vi "9401_UI.vi"(8 "error in (no error)":errorcluster, 11 "Node Ptr":T1 format="%.0x") -> (0 "error out":errorcluster)   [LabVIEW 2019, in "Modules.lvlib" / "9401.lvclass"]
uses:
  9401.lvclass
  <vilib>/NI VeriStand/Custom Device API/Custom Device Item Ref.ctl
  RSI Module/SubPanel Command.ctl
  C:/Users/nitest/Desktop/Git 2019/niveristand-scan-engine-module-libraries/Source/RSI Module/RSI Module.lvclass
  9401.lvclass/9401.ctl
  RSI Module/RSI Module.lvclass
  <vilib>/NI VeriStand/Custom Device API/Custom Device API.lvlib
panel:
  out "_Initial Line Direction Label":string="Initial Line Direction"
  in  "DIO3:0":u32(ring) items=["Input", "Output"]
  in  "DIO7:4":u32(ring) items=["Input", "Output"]
  in  "SubPanel Event":refnum<user-event>
  in  "Header":cluster{"Section Name":string}={"Section Name"="NI 9205 Settings"}
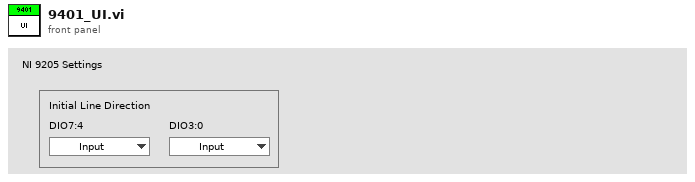
[diagram p1: front panel]
types:
  T1 = typedef "Custom Device API.lvlib/Custom Device Item Ref.ctl" = u64
  T2 = typedef "Modules.lvlib/RSI Module.lvclass/Module Models.ctl" = enum16{"Empty", "NI 9201", "NI 9203", "NI 9205", "NI 9206", "NI 9207", "NI 9208", "NI 9209", "NI 9210", "NI 9211", "NI 9212", "NI 9213", "NI 9214", "NI 9215", "NI 9216", "NI 9217", "NI 9219", "NI 9220", "NI 9221", "NI 9222", "NI 9223", "NI 9224", "NI 9225", "NI 9226", "NI 9227", "NI 9228", "NI 9229", "NI 9233", "NI 9234", "NI 9235", "NI 9236", "NI 9237", "NI 9239", "NI 9242", "NI 9244", "NI 9253", "NI 9263", "NI 9264", "NI 9265", "NI 9266", "NI 9269", "NI 9344", "NI 9350", "NI 9375", "NI 9401", "NI 9402", "NI 9403", "NI 9411", "NI 9421", "NI 9422", "NI 9423", "NI 9425", "NI 9426", "NI 9435", "NI 9436", "NI 9437", "NI 9472", "NI 9474", "NI 9475", "NI 9476", "NI 9477", "NI 9478", "NI 9481", "NI 9482", "NI 9485"}
  T3 = typedef "Modules.lvlib/RSI Module.lvclass/SubPanel Command.ctl" = enum16{"Stop"}
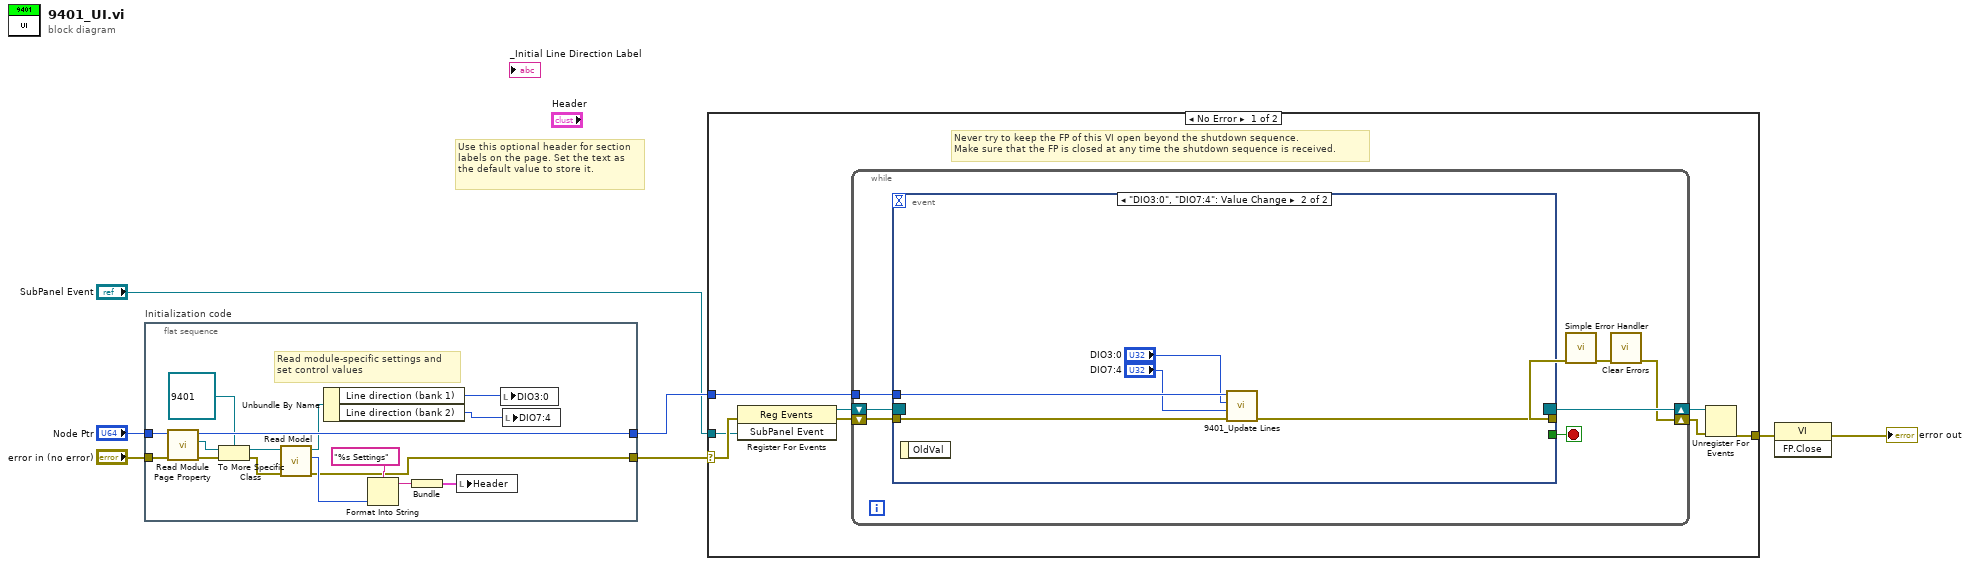
[diagram p0: block diagram]
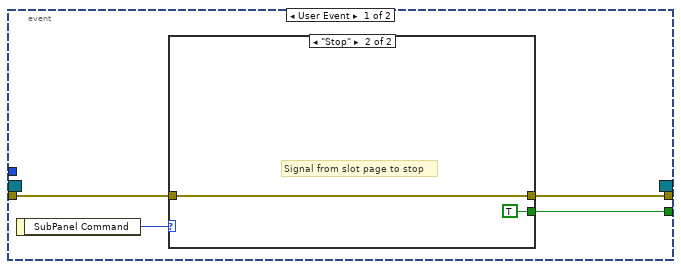
[diagram p2: hidden frame]
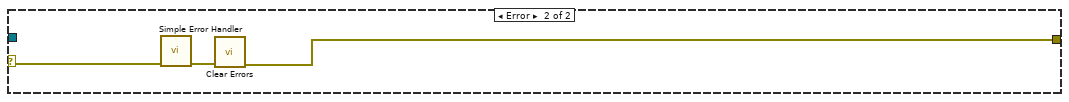
[diagram p4: hidden frame]
diagram:
  # "Use this optional header for section labels on the page. Set the text as the default value to store it."
  n1 = flat-sequence "Initialization code" {
    tunnel: "error in (no error)" -> [w22]
    tunnel: "Node Ptr" -> [w23]
    tunnel: [w10] -> w1
    tunnel: [w21] -> w4
    frame #0 {
      # "Read module-specific settings and\nset control values"
      n2 = call "Read Module Page Property.vi"("error in (no error)"=w22, "Node Ptr In"=w23) -> ("error out"=w20:errorcluster, "RSI Module"=w18:refnum<class "RSI Module.lvclass">, "Node Ptr Out"=w21:T1)  [unwired: 7 in]
      n3 = To More Specific Class(target class=refnum<class "9401.lvclass"> refnum ("9205 in"), reference=w18, error in=w20) -> (specific class reference=w17:refnum<class "9401.lvclass">, error out=w16:errorcluster)
      n4 = call "Read Model.vi"("error in (no error)"=w16, "RSI Module in"=w17) -> ("error out"=w10:errorcluster, "Model"=w14:T2, "RSI Module out"=w11:refnum<class "9401.lvclass">)  [unwired: 7 in]
      n5 = Unbundle By Name(w11) -> ("Line direction (bank 1)"=w9:u32, "Line direction (bank 2)"=w8:u32)
      n6 = Format Into String(format string="%s Settings", w14) -> (resulting string=w12:string)  [unwired: 2 in, 1 out]
      n7 = Bundle(w12) -> (w15:cluster{string})  [unwired: 1 in]
      n8 = local write "Header"(w15) -> ()
      n9 = local write "DIO3:0"(w9) -> ()
      n10 = local write "DIO7:4"(w8) -> ()
    }
  }
  n11 = case shown="No Error" w1 {
    selector: w1 -> [w25 w54]
    tunnel: [w29 w52] -> w7
    tunnel: w4 -> [w26 _]
    tunnel: "SubPanel Event" -> [w24 _]
    frame No Error {
      # "Never try to keep the FP of this VI open beyond the shutdown sequence.\nMake sure that the FP is closed at any time the shutdown sequence is received."
      n12 = register-events(error in=w25, w24) -> (reference out=w27:refnum<event-registration>, error out=w28:errorcluster)  [unwired: 1 in]
      n13 = while {
        tunnel: w26 -> [w35]
        shift-right: [w32] -> w30
        shift-left: w28 -> [w38]
        shift-right: [w39] -> w31
        shift-left: w27 -> [w37]
        stop <- w36 stop-if-true
        n14 = event shown="[1] \"DIO3:0\", \"DIO7:4\": Value Change" {
          selector: w37 -> [_ _]
          dyn-events: [_ _] -> w39
          timeout: _ -> [_ _]
          tunnel: w38 -> [w42 w51]
          tunnel: [w41 _] -> w36
          tunnel: [w40 w50] -> w34
          tunnel: w35 -> [_ w49]
          event User Event {
            n15 = event-data() -> ("SubPanel Command"=w43:T3)  [unwired: 1 out]
            n16 = case shown="\"Stop\"" w43 {
              tunnel: w42 -> [w44 w45]
              tunnel: [w44 w45] -> w40
              tunnel: [_ TRUE] -> w41
              frame Default {
              }
              frame "Stop" {
                # "Signal from slot page to stop"
              }
            }
          }
          event "DIO3:0", "DIO7:4": Value Change {
            n17 = event-data() -> ()  [unwired: 2 out]
            n18 = call "9401_Update Lines.vi"("error in"=w51, "DIO7:4"="DIO7:4", "DIO3:0"="DIO3:0", "Node Ptr in"=w49) -> ("error out"=w50:errorcluster)  [unwired: 6 in, 1 out]
          }
        }
        n19 = call <vilib>:"Simple Error Handler.vi"("error in (no error)"=w34) -> ("error out"=w33:errorcluster)  [unwired: 1 in, 7 out]
        n20 = call <vilib>:"Clear Errors.vi"("error in (no error)"=w33) -> ("error out"=w32:errorcluster)  [unwired: 1 in, 5 out]
      }
      n21 = Unregister For Events(event registration refnum=w31, error in=w30) -> (error out=w29:errorcluster)
    }
    frame Error {
      n22 = call <vilib>:"Simple Error Handler.vi"("error in (no error)"=w54) -> ("error out"=w53:errorcluster)  [unwired: 1 in, 7 out]
      n23 = call <vilib>:"Clear Errors.vi"("error in (no error)"=w53) -> ("error out"=w52:errorcluster)  [unwired: 1 in, 5 out]
    }
  }
  n24 = invoke class="VI" method="FP.Close"(error in=w7) -> (error out=→"error out":errorcluster)  [unwired: 2 in, 2 out]
